vi "GetSutterControllerStatus.vi"() -> ()   [LabVIEW 2014]
uses:
  SerialController/Serial Controller.lvclass
panel:
  in  "Stop":bool
  out "Multiplier msteps/mm":u16
  out "Divisor msteps/mm":u16
  out "Adjusted Pulse Speed":u16
  out "Microsteps Per Pulse":u16
  out "Velocity mm/s":u16
  out "Firmware Version":u16
  out "Hi Resolution":bool
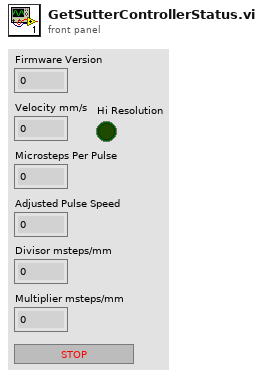
[diagram p1: front panel]
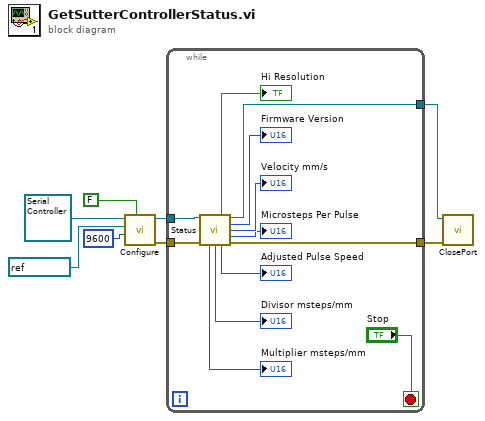
[diagram p0: block diagram]
diagram:
  n1 = call-dynamic "Configure.vi"("Reset"=FALSE, "baud rate (9600)"=u32 9600, "VISA resource name"=refnum<visa-resource-name> "COM3", "Serial Controller in"=refnum<class "Serial Controller.lvclass"> refnum) -> ("error out"=w3:errorcluster, "Serial Controller out"=w4:refnum<class "Serial Controller.lvclass">)  [unwired: 6 in]
  n2 = while {
    tunnel: w4 -> [w20]
    tunnel: w3 -> [w19]
    tunnel: [w17] -> w2
    tunnel: [w18] -> w1
    stop <- "Stop" stop-if-true
    n3 = call-dynamic "Status.vi"("Serial Controller in"=w20, "error in (no error)"=w19) -> ("Hi Resolution"=→"Hi Resolution":bool, "Serial Controller out"=w17:refnum<class "Serial Controller.lvclass">, "Firmware Version"=→"Firmware Version":u16, "Velocity mm/s"=→"Velocity mm/s":u16, "Microsteps Per Pulse"=→"Microsteps Per Pulse":u16, "Multiplier msteps/mm"=→"Multiplier msteps/mm":u16, "Divisor msteps/mm"=→"Divisor msteps/mm":u16, "Adjusted Pulse Speed"=→"Adjusted Pulse Speed":u16, "error out"=w18:errorcluster)  [unwired: 5 in]
  }
  n4 = call-dynamic "ClosePort.vi"("error in (no error)"=w1, "Serial Controller in"=w2) -> ()  [unwired: 9 in, 1 out]
